vi "Read Registered Views.vi"(0 "Controller Actor in":refnum<class "Controller Actor.lvclass">, 5 "error in (no error)":errorcluster) -> (14 "Controller Actor out":refnum<class "Controller Actor.lvclass">, 19 "error out":errorcluster)   [LabVIEW 2023, in "Event Actors.lvlib" / "Controller Actor.lvclass"]
doc: "Allows the child controller to read the registered views by registering to the user defined event whose reference is accessible by the <b>Registered Views Event Ref</b> property"
uses:
  Controller Actor.lvclass
  Controller Actor.lvclass/Controller Actor.ctl
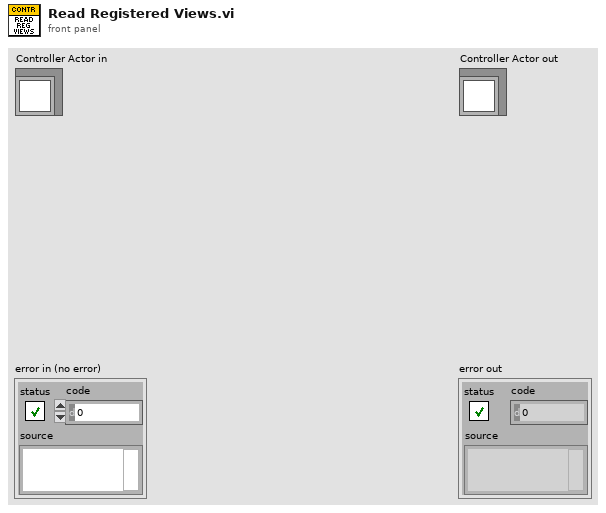
[diagram p1: front panel]
types:
  T1 = typedef "Event Actors.lvlib/Controller Actor.lvclass/Registered Views Event Ref.ctl" = refnum<user-event>
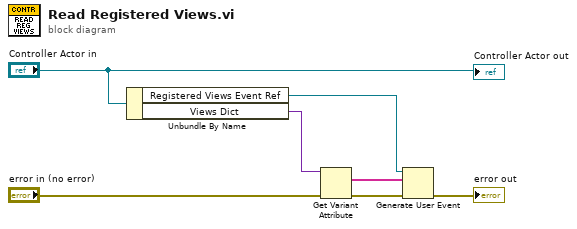
[diagram p0: block diagram]
diagram:
  n1 = Unbundle By Name("Controller Actor in") -> ("Registered Views Event Ref"=w2:T1, "Views Dict"=w7:variant)
  n2 = Get Variant Attribute(Variant=w7, error in="error in (no error)") -> (names=w1:string[], error out=w4:errorcluster)  [unwired: 2 in, 2 out]
  n3 = Generate User Event(user event=w2, event data cluster=w1, error in=w4) -> (error out=→"error out":errorcluster)  [unwired: 1 in, 1 out]
  "Controller Actor out" <- "Controller Actor in"
